vi "LTC20 change temp v0.3.vi"(3 "LTC-GPIB\nAddress":refnum<visa-resource-name>) -> (0 "Stop":bool, 1 "Stable Temperature (K)":dbl format="%.2f")   [LabVIEW 2024]
doc: "Changes the setpoint and waits for temperature to stablilize near the setpoint. Can set how stable and how close to the setpoint one wants the temperature to be. Allows changing of the PID parameters.\nMurali Chaparala, Scott Hannahs, NHMFL - FSU, November 1996"
uses:
  <vilib>/Analysis/NI_AALBase.lvlib
panel:
  out "Current Temperature Profile":dbl[](graph)=[0.0, 0.0, 0.0, 0.0, 0.0, 0.0, 0.0, 0.0, 0.0, 0.0, 0.0, 0.0, 0.0, 0.0, 0.0, 0.0, 0.0, 0.0, 0.0, 0.0, nan, nan, nan, nan, nan, nan, nan, nan, nan, nan, nan, nan, nan, nan, nan, nan, nan, nan, nan, nan, nan, nan, nan, nan, nan, nan, nan, nan, nan, nan, nan, nan, nan, nan, nan, nan, nan, nan, nan, nan]
  in  "PID param":dbl[][](array[numeric])=[[1.0, 0.0, 0.0, 0.0], [1.0, 0.0, 0.0, 0.0]] format="%.3f"
  out "Temperature set points":dbl[](array[numeric]) format="%.2f"
  in  "File containing the temperature set points:":path
  in  "Use Sensor 2?":bool
  out "Stable temperature (K)":dbl[](array[numeric]) format="%.2f"
  in  "Difference between\nInner and outer temperature (K).":dbl=3.0 min=0.0 max=20.0 step=1.0 format="%.2f"
  in  "Number of data sets to read for each stable temperature?":i32=10 min=1 step=1
  in  "Point Number":i32 min=-20 step=1
  in  "What is the % deviation\nof the STABLE, AVERAGE \nsample  temperature from\nthe set point that we \nconsider acceptable?":dbl=0.05000000000000002 min=0.0 max=100.0 step=0.01 format="%.3f"
  in  "What is the % variation of\nthe sample temperature \nabout the mean value that\nwe consider acceptable to\ndefine it as being stable?":dbl=0.01000000000000001 min=0.0 max=100.0 step=0.01 format="%.3f"
  in  "Number of points\nused to determine \nstable temperature.":i32=60 min=1 max=1000 step=1
  in  "DeltaT (ms)":u32=1000 max=3600000 step=10
  out "Time over which the stability\ncriterion was satisfied (S).":dbl=18.933 format="%.2f"
  out "Temperature Fluctuation \nabout the AVERAGE \nvalue (%).":dbl min=0.0 format="%.3f"
  out "% Deviation of the\nsample temperature\nfrom the set point.":dbl=0.001 min=0.001 max=310.0 format="%.3f"
  # "Sensor1 Panel"
  # "Sensor 2 Panel"
  # "Stability Panel"
  # "Heater"
  # "Analog"
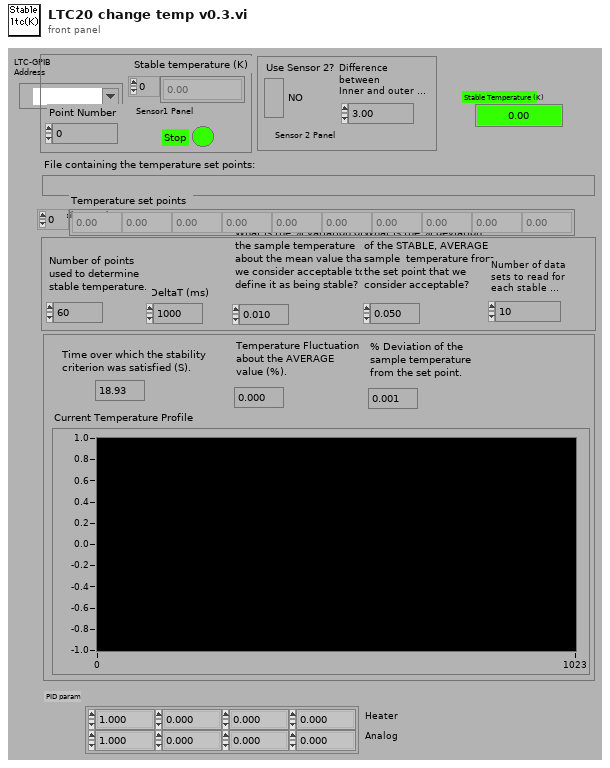
[diagram p1: front panel]
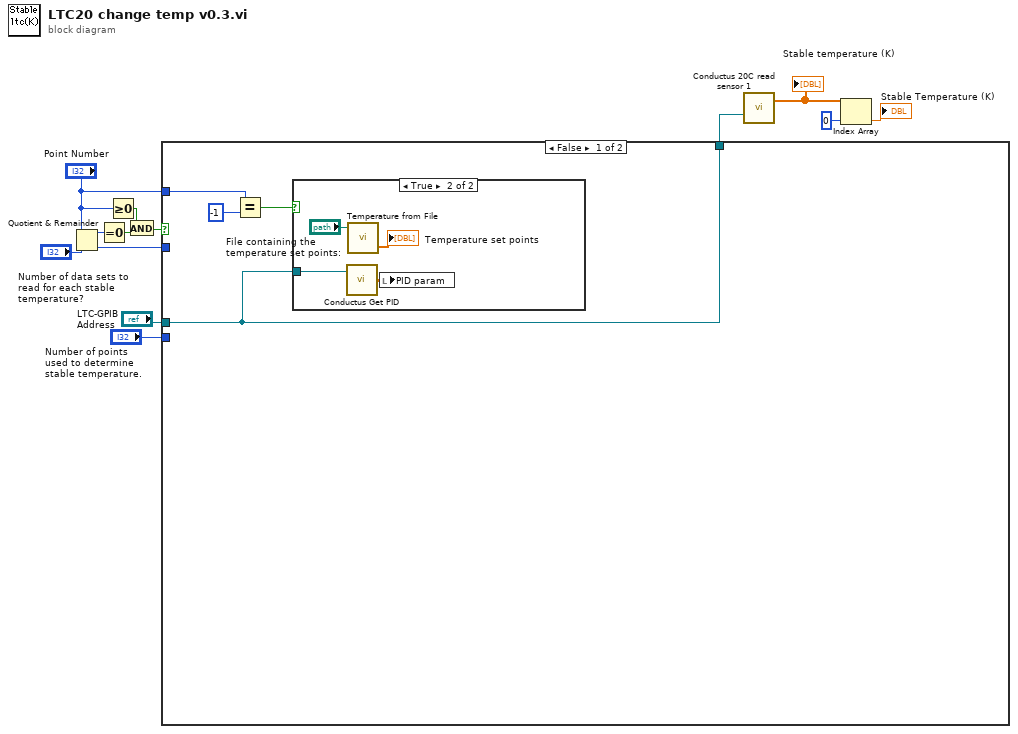
[diagram p0: block diagram]
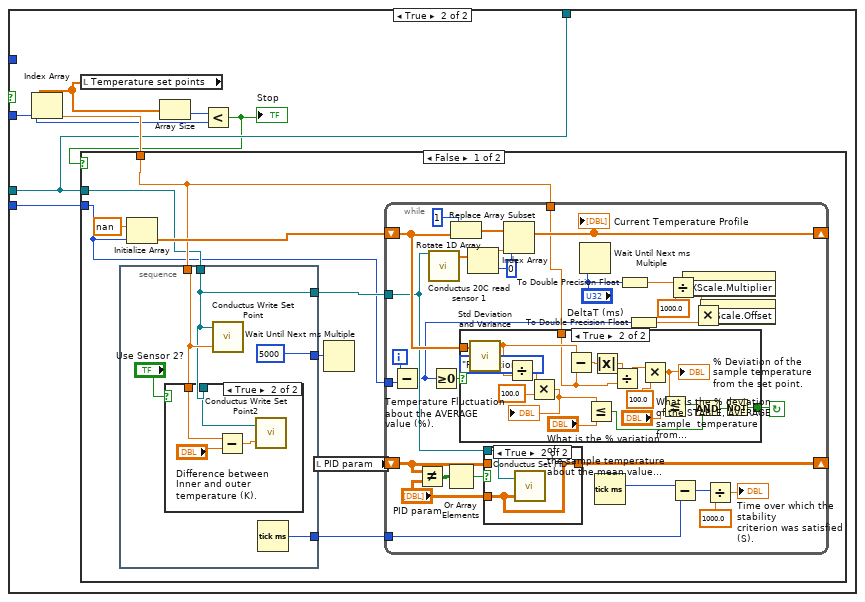
[diagram p3: hidden frame]
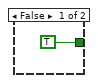
[diagram p5: hidden frame]
diagram:
  n1 = Quotient & Remainder(x="Point Number", y="Number of data sets to read for each stable temperature?") -> (x-y*floor(x/y)=w13:i32, floor(x/y)=w10:i32)
  n2 = Equal To 0?(x=w13) -> (x = 0?=w8:bool)
  n3 = Greater Or Equal To 0?(x="Point Number") -> (x >= 0?=w9:bool)
  n4 = And(x=w9, y=w8) -> (x .and. y?=w7:bool)
  n5 = case shown="False" w7 {
    tunnel: "LTC-GPIB\nAddress" -> [w14 w26]
    tunnel: "Number of points\nused to determine \nstable temperature." -> [_ w27]
    tunnel: w10 -> [_ w23]
    tunnel: [w14 w26] -> w6
    tunnel: "Point Number" -> [w16 _]
    frame False {
      n6 = Equal?(x=w16, y=-1) -> (x = y?=w15:bool)
      n7 = case shown="True" w15 {
        tunnel: w14 -> [_ w19]
        frame False {
        }
        frame True {
          n8 = call "Conductus Get PID.vi"("Instrument Address"=w19) -> ("PID Param"=w18:dbl[][])  [unwired: 1 in, 1 out]
          n9 = call "Temperature from File.vi"("File Name:"="File containing the temperature set points:") -> ("Temperature set points"=→"Temperature set points":dbl[])  [unwired: 1 out]
          n10 = local write "PID param"(w18) -> ()
        }
      }
    }
    frame True {
      n11 = local read "Temperature set points"() -> (w25:dbl[])
      n12 = Index Array(array=w25, index=w23) -> (element=w28:dbl)
      n13 = Array Size(array=w25) -> (size(s)=w24:i32)
      n14 = Less?(x=w24, y=w23) -> (x < y?=w22:bool)
      "Stop" <- w22
      n15 = case shown="False" w22 {
        tunnel: w28 -> [w35 _]
        tunnel: w26 -> [w32 _]
        tunnel: w27 -> [w31 _]
        frame False {
          n16 = stacked-sequence {
            tunnel: w32 -> [w92]
            tunnel: w35 -> [w95]
            tunnel: [u32 5000] -> w34
            tunnel: [w92] -> w33
            tunnel: [w91] -> w29
            frame #0 {
              n17 = case shown="True" "Use Sensor 2?" {
                tunnel: w95 -> [_ w98]
                tunnel: w92 -> [_ w96]
                frame False {
                }
                frame True {
                  n18 = Subtract(x=w98, y="Difference between\nInner and outer temperature (K).") -> (x-y=w97:dbl)
                  n19 = call "Conductus Write Set Point2.vi"("Setpoint"=w97, "GPIB Address"=w96) -> ()  [unwired: 1 in]
                }
              }
              n20 = call "Conductus Write Set Point.vi"("Setpoint"=w95, "Instrument Address"=w92) -> ()  [unwired: 1 in]
              n21 = Tick Count (ms)() -> (millisecond timer value=w91:u32)
            }
          }
          n22 = Initialize Array(nan, w31) -> (w37:dbl[])
          n23 = local read "PID param"() -> (w30:dbl[][])
          n24 = Wait Until Next ms Multiple(millisecond multiple=w34) -> ()  [unwired: 1 out]
          n25 = while {
            tunnel: w29 -> [w46]
            shift-left: w30 -> [w51]
            shift-right: [w50] -> _
            tunnel: w33 -> [w49]
            tunnel: w35 -> [w57]
            tunnel: w31 -> [w61]
            shift-left: w37 -> [w58]
            shift-right: [w62] -> _
            i -> [w60]
            stop <- w59 continue-if-true
            w66 = 0
            n26 = Subtract(x=w60, y=w61) -> (x-y=w42:i32)
            n27 = Not Equal?(x=w51, y="PID param") -> (x != y?=w53:bool[][])
            n28 = call "Conductus 20C read sensor 1.vi"("Instrument Address"=w49) -> ("Output"=w65:dbl[])  [unwired: 1 in, 1 out]
            n29 = Greater Or Equal To 0?(x=w42) -> (x >= 0?=w43:bool)
            n30 = Or Array Elements(Boolean array=w53) -> (logical OR=w52:bool)
            n31 = Rotate 1D Array(1:w58, 2:1) -> (0:w64:dbl[])
            n32 = case shown="True" w43 {
              tunnel: [TRUE w73] -> w59
              tunnel: w58 -> [_ w75]
              tunnel: w57 -> [_ w74]
              frame False {
              }
              frame True {
                n33 = call <vilib>:"Std Deviation and Variance.vi"("X"=w75, "Weighting (Sample)"=enum16{"Sample", "Population"}."Population") -> ("mean"=w88:dbl, "standard deviation"=w87:dbl)  [unwired: 1 out]
                n34 = Divide(x=w87, y=w88) -> (x/y=w81:dbl)
                n35 = Multiply(x=w81, y=100.0) -> (x*y=w89:dbl)
                "Temperature Fluctuation \nabout the AVERAGE \nvalue (%)." <- w89
                n36 = Subtract(x=w88, y=w74) -> (x-y=w76:dbl)
                n37 = Less Or Equal?(x=w89, y="What is the % variation of\nthe sample temperature \nabout the mean value that\nwe consider acceptable to\ndefine it as being stable?") -> (x <= y?=w84:bool)
                n38 = Absolute Value(x=w76) -> (abs(x)=w77:dbl)
                n39 = Divide(x=w77, y=w74) -> (x/y=w78:dbl)
                n40 = Multiply(x=w78, y=100.0) -> (x*y=w86:dbl)
                "% Deviation of the\nsample temperature\nfrom the set point." <- w86
                n41 = Less Or Equal?(x=w86, y="What is the % deviation\nof the STABLE, AVERAGE \nsample  temperature from\nthe set point that we \nconsider acceptable?") -> (x <= y?=w90:bool)
                n42 = And(x=w90, y=w84) -> (x .and. y?=w85:bool)
                n43 = Not(x=w85) -> (.not. x?=w73:bool)
              }
            }
            n44 = Index Array(array=w65, index=w66) -> (element=w67:dbl)
            n45 = case shown="True" w52 {
              tunnel: "PID param" -> [_ w70]
              tunnel: [w68 w70] -> w50
              tunnel: w51 -> [w68 _]
              tunnel: w49 -> [_ w69]
              frame False {
              }
              frame True {
                n46 = call "Conductus Set PID.vi"("PID param"=w70, "Instrument Address"=w69) -> ()  [unwired: 1 in, 1 out]
              }
            }
            n47 = Replace Array Subset(array=w64, new element=w67, index=w66) -> (w62:dbl[])
            "Current Temperature Profile" <- w62
            n48 = Wait Until Next ms Multiple(millisecond multiple="DeltaT (ms)") -> ()  [unwired: 1 out]
            n49 = Tick Count (ms)() -> (millisecond timer value=w44:u32)
            n50 = To Double Precision Float(number="DeltaT (ms)") -> (double precision float=w38:dbl)
            n51 = To Double Precision Float(number=w42) -> (double precision float=w39:dbl)
            n52 = Divide(x=w38, y=1000.0) -> (x/y=w41:dbl)
            n53 = Subtract(x=w44, y=w46) -> (x-y=w45:u32)
            n54 = property on="Current Temperature Profile" class="WFChart (strict)"("XScale.Multiplier"=w41) -> ()  [unwired: 2 in, 2 out]
            n55 = Multiply(x=w41, y=w39) -> (x*y=w40:dbl)
            n56 = property on="Current Temperature Profile" class="WFChart (strict)"("XScale.Offset"=w40) -> ()  [unwired: 2 in, 2 out]
            n57 = Divide(x=w45, y=1000.0) -> (x/y=→"Time over which the stability\ncriterion was satisfied (S).":dbl)
          }
        }
        frame True {
        }
      }
    }
  }
  n58 = call "Conductus 20C read sensor 1.vi"("Instrument Address"=w6) -> ("Output"=w2:dbl[])  [unwired: 1 in, 1 out]
  "Stable temperature (K)" <- w2
  n59 = Index Array(array=w2, index=0) -> (element=→"Stable Temperature (K)":dbl)
